vi "Wrapper.vi"(0 "Current Setpoint":dbl, 5 "Voltage Setpoint":dbl, 7 "Physical Channel":tag, 9 "Calculate Analysis?":bool, 11 "error in (no error)":errorcluster) -> (4 "voltage":dbl[](array[numeric]), 6 "Current":dbl[](array[numeric]), 15 "error out":errorcluster)   [LabVIEW 2021, in "Power Measurement.lvlib"]
uses:
  Typedefs/Pow Meas Init Settings.ctl
  Typedefs/Pow Meas Timing Settings.ctl
  Typedefs/Pow Meas Rigger Settings.ctl
  Typedefs/pow Meas Configure or Measure.ctl
  Power Measurement.lvlib
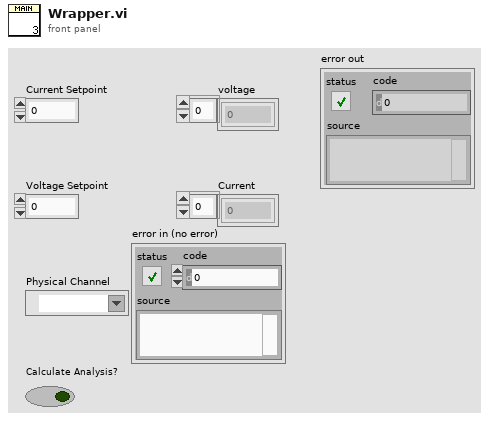
[diagram p1: front panel]
types:
  T1 = typedef "Power Measurement.lvlib/pow Meas Configure or Measure.ctl" = enum16{"Configure Only", "Measure Only", "Configure and Measure"}
  T2 = typedef "Power Measurement.lvlib/Pow Meas Rigger Settings.ctl" = cluster{"Digital Start Trigger?":bool, "Digital Start Trigger Source":tag, "Digital Start Trigger Edge":i32}
  T3 = typedef "Power Measurement.lvlib/Pow Meas Timing Settings.ctl" = cluster{"Sample Clock Source":tag, "Sample Rate":dbl, "Number of Samples":i32}
  T4 = typedef "Power Measurement.lvlib/Pow Meas Init Settings.ctl" = cluster{"Current Setpoint":dbl, "Voltage Setpoint":dbl}
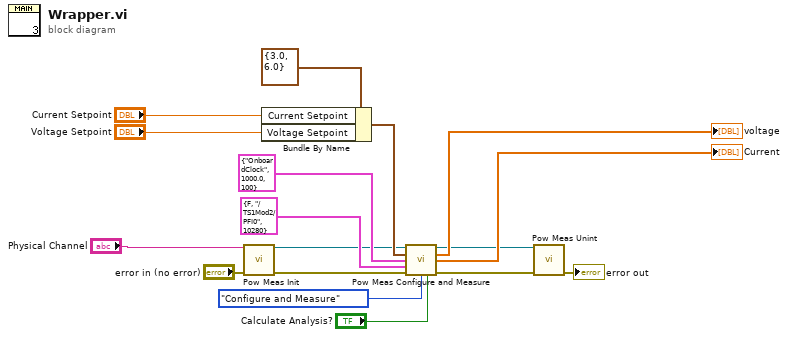
[diagram p0: block diagram]
diagram:
  n1 = call "Pow Meas Init.vi"("Physical Channel"="Physical Channel", "error in (no error)"="error in (no error)") -> ("task out"=w3:refnum<k21>, "error out"=w4:errorcluster)  [unwired: 12 in]
  n2 = Bundle By Name(cluster=T4 {"Current Setpoint"=3.0, "Voltage Setpoint"=6.0} ("Channel Settings"), "Current Setpoint"="Current Setpoint", "Voltage Setpoint"="Voltage Setpoint") -> (w13:T4)
  n3 = call "Pow Meas Configure and Measure.vi"("task/channels in"=w3, "Channel Settings"=w13, "Timing Settings"=T3 {"Sample Clock Source"="OnboardClock", "Sample Rate"=1000.0, "Number of Samples"=100}, "Trigger Settings"=T2 {"Digital Start Trigger?"=FALSE, "Digital Start Trigger Source"="/TS1Mod2/PFI0", "Digital Start Trigger Edge"=10280}, "error in (no error)"=w4, "Operation"=pow_Meas_Configure_or_Measure."Configure and Measure", "Calculate Analysis?"="Calculate Analysis?") -> ("task out"=w6:refnum<k21>, "voltage"=→"voltage":dbl[], "Current"=→"Current":dbl[], "error out"=w7:errorcluster)  [unwired: 4 in, 1 out]
  n4 = call "Pow Meas Unint.vi"("task/channels in"=w6, "error in (no error)"=w7) -> ("error out"=→"error out":errorcluster)  [unwired: 13 in]
